vi "Measurement UI.vi"() -> ()   [LabVIEW 2021, in "Quiescent Current_PMIC_UI.lvlib"]
uses:
  Quiescent Current_PMIC_UI.lvlib
panel:
  in  "MeasGraphs":enum32{"Q Current", "Hidden Controls"}(tab)
  out "QCurrentGraph(V/A)":T1(graph)
  out "Q current minimum":dbl
  out "Q current maximum":dbl
  out "Q currents":dbl[](array[numeric])
  out "Source voltages":dbl[](array[numeric])
  in  "Source resource name":string
  out "MeasTable":string[][](table)
  in  "Source sense":i32(ring)=1009 caption="SENSE" items=["Local"=1008, "Remote"=1009]
  in  "PPSResourceName":refnum<k15> caption="RESOURCE NAME"
  in  "DUT setup time":dbl=1.0 caption="DUT SETUP TIME" format="%#_6ps"
  in  "Source stop voltage":dbl=20.0 caption="STOP VOLTAGE" format="%#_6pV"
  in  "Source start voltage":dbl=6.0 caption="START VOLTAGE" format="%#_6pV"
  in  "Source voltage sweep points":i32=10 caption="SWEEP POINTS"
  in  "Aperture time":dbl=0.005 caption="APERTURE TIME" format="%#_6ps"
  in  "Source delay":dbl=0.005 caption="SOURCE DELAY" format="%#_6ps"
  in  "Source current limit":dbl=25.0 caption="CURRENT LIMIT" format="%#_6pA"
  in  "Source maximum power":dbl=300.0 caption="MAXIMUM POWER" format="%#_6pW"
  in  "Source configuration":string="Source configuration"
  in  "Measurement settings":string="Measurement settings"
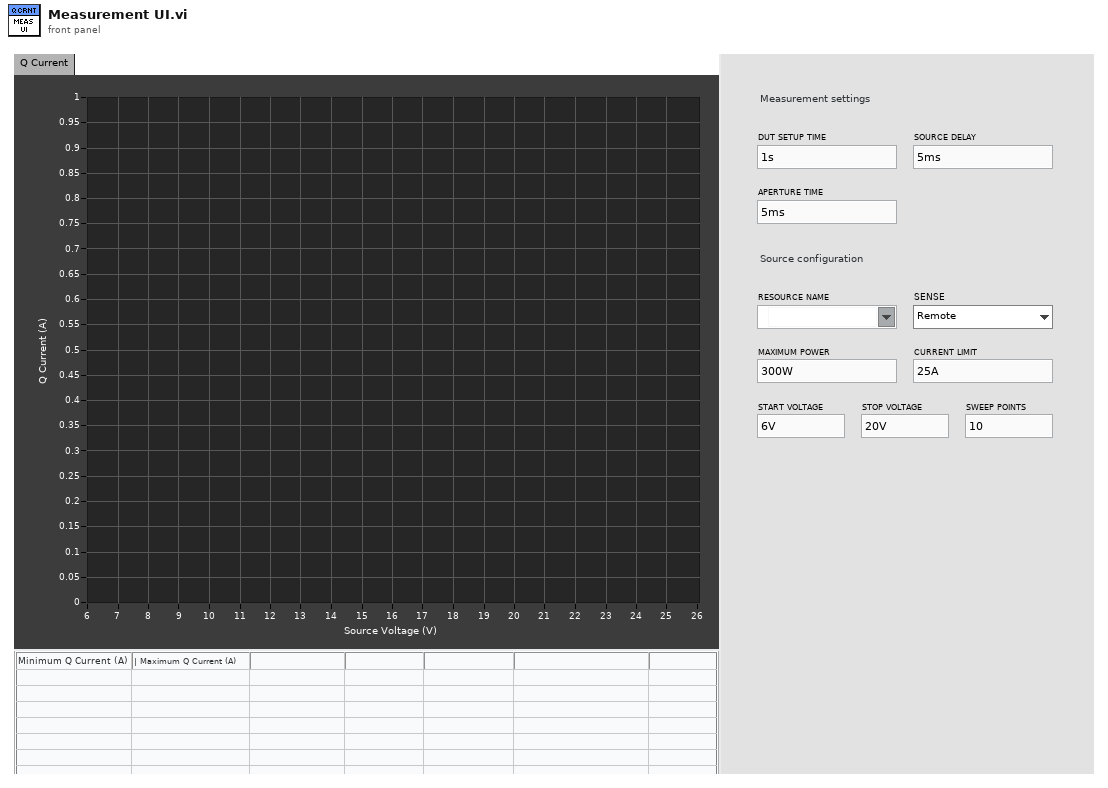
[diagram p1: front panel]
types:
  T1 = cluster{"Source voltages":dbl[], "Load voltages":dbl[]}
  T2 = cluster{"Source voltages":dbl[], "Q currents":dbl[]}
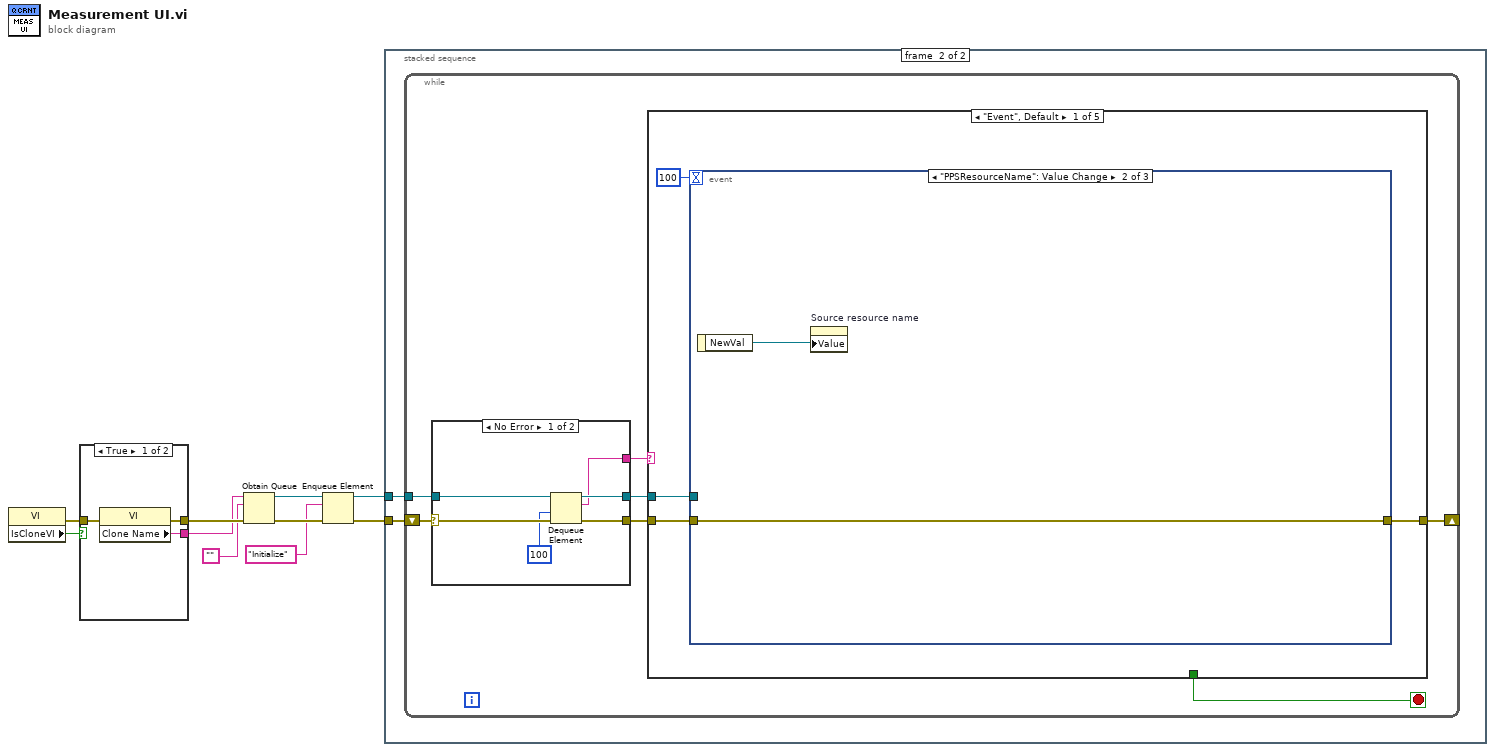
[diagram p0: block diagram]
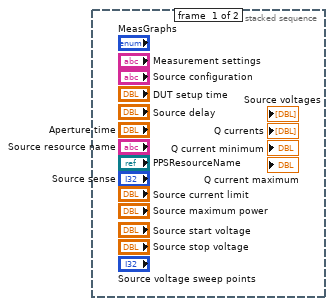
[diagram p2: hidden frame]
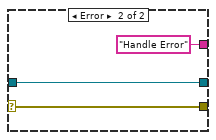
[diagram p3: hidden frame]
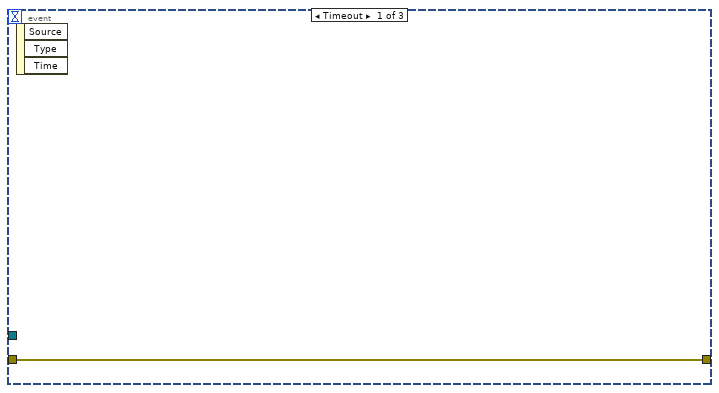
[diagram p4: hidden frame]
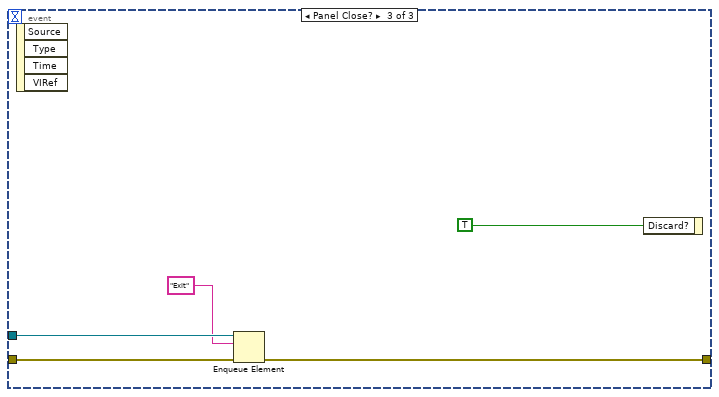
[diagram p5: hidden frame]
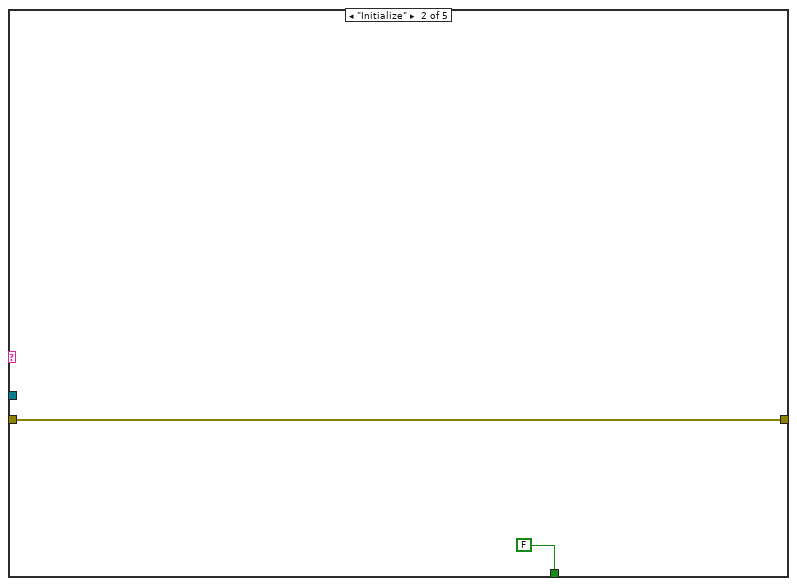
[diagram p6: hidden frame]
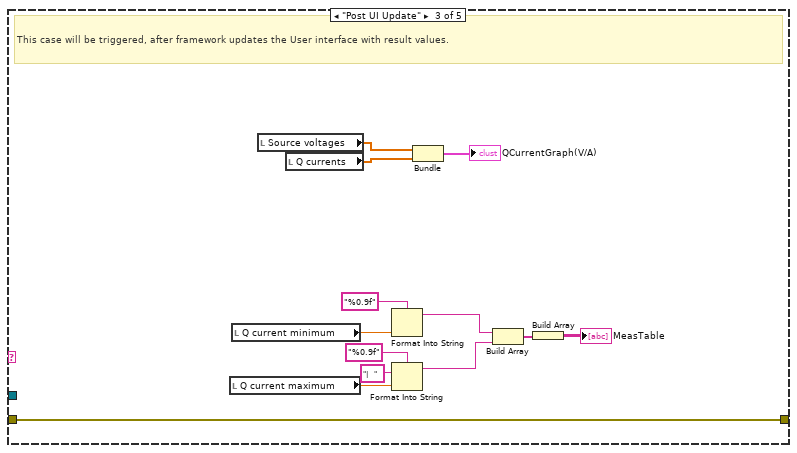
[diagram p7: hidden frame]
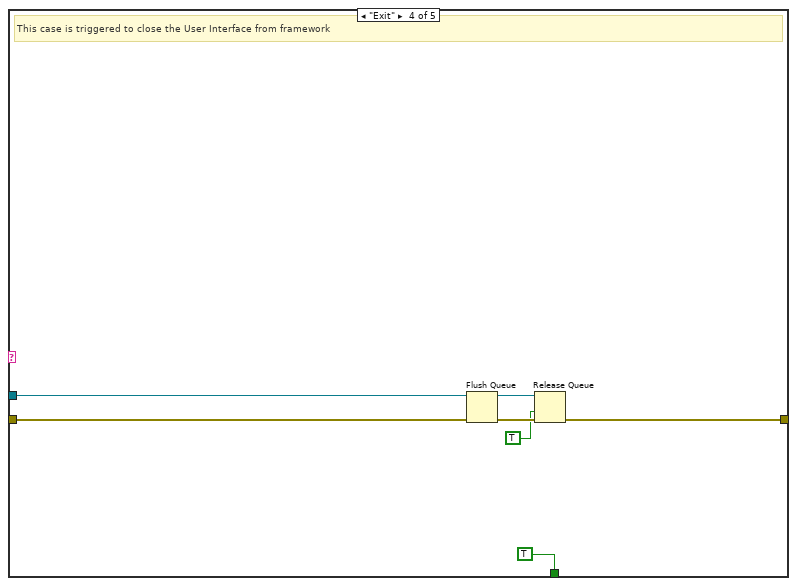
[diagram p8: hidden frame]
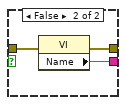
[diagram p10: hidden frame]
diagram:
  n1 = property class="VI"() -> (error out=w1:errorcluster, "IsCloneVI"=w2:bool)  [unwired: 2 in, 1 out]
  n2 = case shown="True" w2 {
    tunnel: [w13 w16] -> w10
    tunnel: [w12 w15] -> w9
    tunnel: w1 -> [w11 w14]
    frame True {
      n3 = property class="VI"(error in=w11) -> (error out=w13:errorcluster, "Clone Name"=w12:string)  [unwired: 1 in, 1 out]
    }
    frame False {
      n4 = property class="VI"(error in=w14) -> (error out=w16:errorcluster, "Name"=w15:string)  [unwired: 1 in, 1 out]
    }
  }
  n5 = Obtain Queue(name (unnamed)=w9, element data type="", error in (no error)=w10) -> (queue out=w6:refnum<queue>, error out=w8:errorcluster)  [unwired: 2 in, 1 out]
  n6 = Enqueue Element(queue=w6, element="Initialize", error in (no error)=w8) -> (queue out=w5:refnum<queue>, error out=w7:errorcluster)  [unwired: 1 in, 1 out]
  n7 = stacked-sequence {
    tunnel: w7 -> [_ w18]
    tunnel: w5 -> [_ w17]
    frame #0 {
    }
    frame #1 {
      n8 = while {
        shift-right: [w20] -> _
        shift-left: w18 -> [w25]
        tunnel: w17 -> [w23]
        stop <- w19 stop-if-true
        n9 = case shown="No Error" w25 {
          selector: w25 -> [w31 w34]
          tunnel: [w30 w34] -> w24
          tunnel: w23 -> [w29 w33]
          tunnel: [w28 w33] -> w22
          tunnel: [w27 "Handle Error"] -> w21
          frame No Error {
            n10 = Dequeue Element(queue=w29, timeout in ms (-1)=100, error in (no error)=w31) -> (queue out=w28:refnum<queue>, element=w27:string, error out=w30:errorcluster)  [unwired: 1 out]
          }
          frame Error {
          }
        }
        n11 = case shown="\"Event\", Default" w21 {
          tunnel: w24 -> [w37 w48 w61 w68 w69]
          tunnel: w22 -> [w35 _ _ w66 _]
          tunnel: [w38 w48 w61 w63 w69] -> w20
          tunnel: [_ FALSE _ TRUE _] -> w19
          frame "Event", Default {
            n12 = event shown="[1] \"PPSResourceName\": Value Change" {
              selector: _ -> [_ _ _]
              dyn-events: _ -> [_ _ _]
              timeout: 100 -> [_ _ _]
              tunnel: [w39 w40 w44] -> w38
              tunnel: w37 -> [w39 w40 w45]
              tunnel: w35 -> [_ _ w43]
              event Timeout {
                n13 = event-data() -> ()  [unwired: 1 in, 3 out]
              }
              event "PPSResourceName": Value Change {
                n14 = event-data() -> ("NewVal"=w41:refnum<k15>)  [unwired: 1 in]
                n15 = property on="Source resource name" class="Str"("Value"=w41) -> ()  [unwired: 2 in, 2 out]
              }
              event Panel Close? {
                n16 = event-data() -> ()  [unwired: 1 in, 4 out]
                n17 = Enqueue Element(queue=w43, element="Exit", error in (no error)=w45) -> (error out=w44:errorcluster)  [unwired: 1 in, 2 out]
                n18 = event-data("Discard?"=TRUE) -> ()  [unwired: 1 in, 1 out]
              }
            }
          }
          frame "Initialize" {
          }
          frame "Post UI Update" {
            # "This case will be triggered, after framework updates the User interface with result values."
            n19 = local read "Q current maximum"() -> (w54:dbl)
            n20 = local read "Q current minimum"() -> (w55:dbl)
            n21 = local read "Source voltages"() -> (w60:dbl[])
            n22 = local read "Q currents"() -> (w59:dbl[])
            n23 = Format Into String(format string="%0.9f" ("initial string"), w55) -> (resulting string=w53:string)  [unwired: 2 in, 1 out]
            n24 = Format Into String(format string="%0.9f" ("initial string"), initial string="|   ", w54) -> (resulting string=w52:string)  [unwired: 1 in, 1 out]
            n25 = Bundle("Source voltages"=w60, "Q currents"=w59) -> (→"QCurrentGraph(V/A)":T2)  [unwired: 1 in]
            n26 = Build Array(w53, w52) -> (w51:string[])
            n27 = Build Array(w51) -> (→"MeasTable":string[][])
          }
          frame "Exit" {
            # "This case is triggered to close the User Interface from framework"
            n28 = Flush Queue(queue=w66, error in (no error)=w68) -> (queue out=w65:refnum<queue>, error out=w64:errorcluster)  [unwired: 1 out]
            n29 = Release Queue(queue=w65, force destroy? (F)=TRUE, error in (no error)=w64) -> (error out=w63:errorcluster)  [unwired: 2 out]
          }
          frame "Handle Error" {
          }
        }
      }
    }
  }
